vi "prueba5lector.vi"() -> ()   [LabVIEW 2012]
panel:
  out "Array":T1(array[cluster]) {"tanque3" scale=0.0..10.0; "tanque2" scale=0.0..10.0; "tanque1" scale=0.0..10.0}
  # "Elaborar un programa para adicionar este cluster a un archivo de texto.\nLuego debera hacer otro programa donde lea la informacion del archivo \nde texto y lo coloque en el cluster."
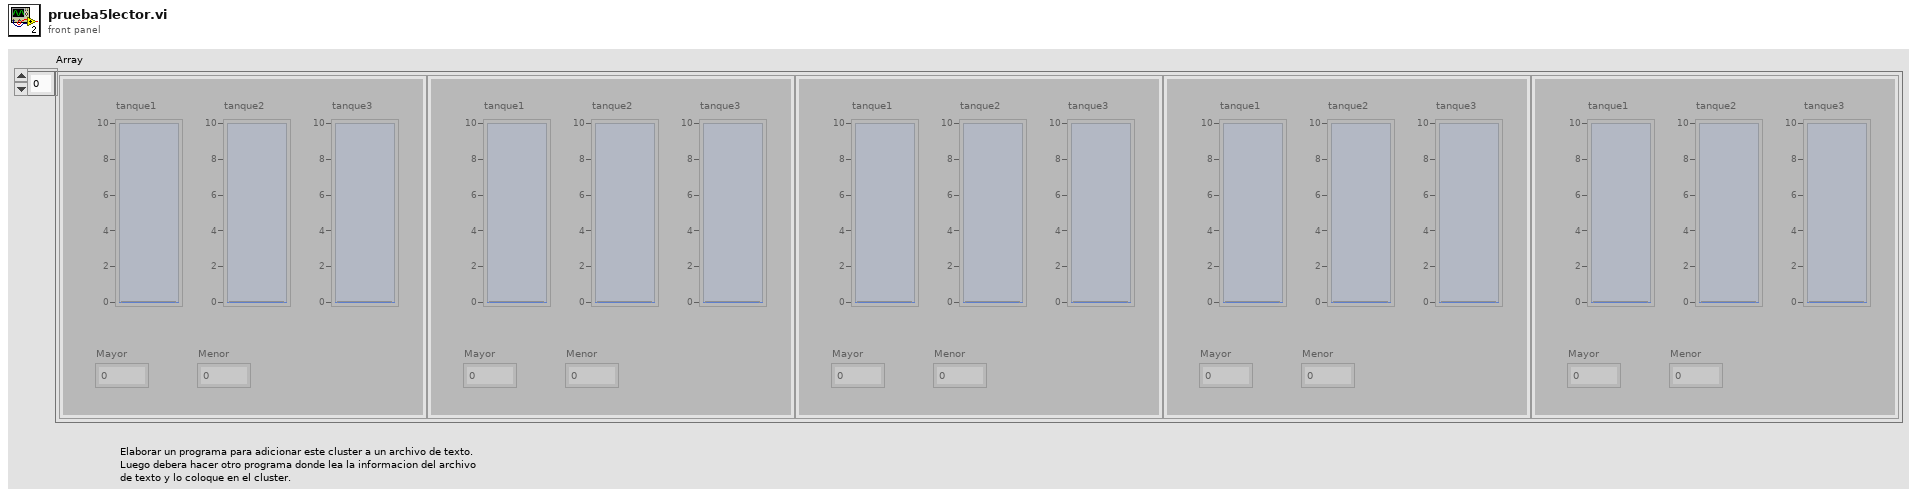
[diagram p1: front panel]
types:
  T1 = cluster{"tanque1":i32, "tanque2":i32, "tanque3":i32, "Mayor":dbl, "Menor":dbl}[]
  T2 = enum16{"open", "replace", "create", "open or create", "replace or create", "replace or create with confirmation"}
  T3 = cluster{"tanque1":i32, "tanque2":i32, "tanque3":i32, "Mayor":dbl, "Menor":dbl}
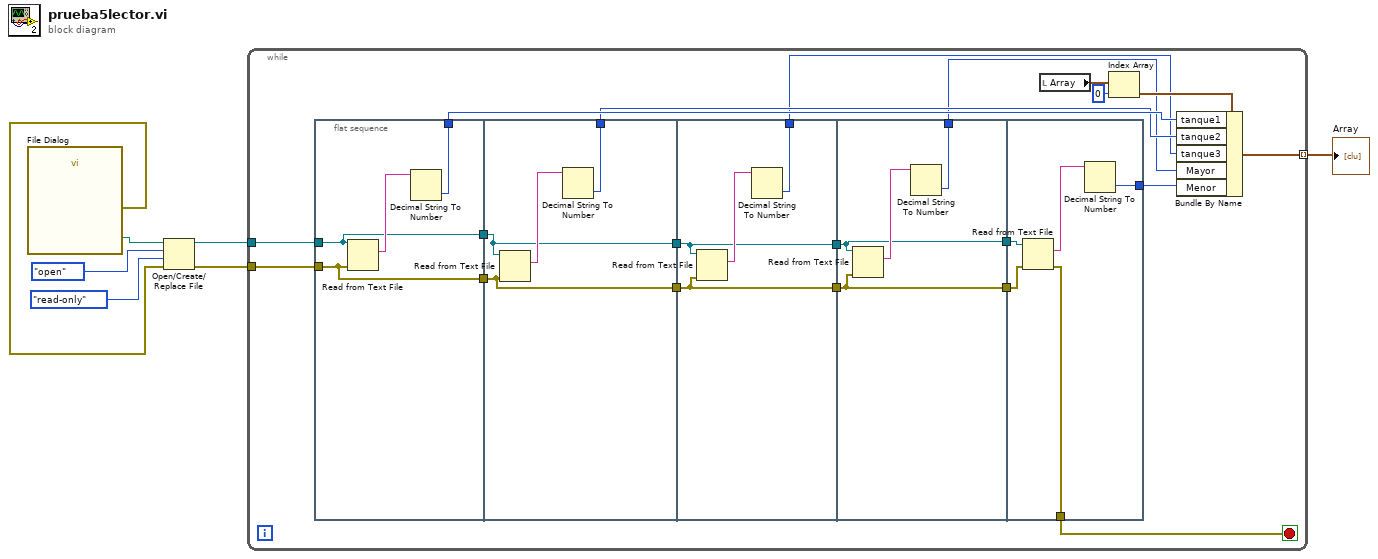
[diagram p0: block diagram]
diagram:
  n1 = call "File Dialog"() -> ("selected path"=w7:path, "error out"=w6:errorcluster)  [unwired: 12 in, 2 out]
  n2 = Open/Create/Replace File(file path (use dialog)=w7, error in=w6, operation (0:open)=T2."open", access (0:read/write)=enum16{"read/write", "read-only", "write-only"}."read-only") -> (refnum out=w3:refnum<file>, error out=w2:errorcluster)  [unwired: 2 in, 1 out]
  n3 = while {
    tunnel: w3 -> [w27]
    tunnel: w2 -> [w26]
    tunnel: [w8] -> w1 mode=indexing
    stop <- w17 stop-if-true
    n4 = flat-sequence {
      tunnel: w27 -> [w29]
      tunnel: w26 -> [w30]
      tunnel: [w30] -> w25
      tunnel: [w29] -> w24
      tunnel: [w28] -> w13
      tunnel: w25 -> [w34]
      tunnel: w24 -> [w33]
      tunnel: [w34] -> w23
      tunnel: [w33] -> w22
      tunnel: [w32] -> w12
      tunnel: w23 -> [w38]
      tunnel: w22 -> [w37]
      tunnel: [w38] -> w21
      tunnel: [w37] -> w20
      tunnel: [w36] -> w11
      tunnel: w21 -> [w42]
      tunnel: w20 -> [w41]
      tunnel: [w42] -> w19
      tunnel: [w41] -> w18
      tunnel: [w40] -> w10
      tunnel: w19 -> [w48]
      tunnel: w18 -> [w47]
      tunnel: [w45] -> w17
      tunnel: [w44] -> w9
      frame #0 {
        n5 = Read from Text File(file (use dialog)=w29, error in=w30) -> (text=w31:string)  [unwired: 2 in, 3 out]
        n6 = Decimal String To Number(string=w31) -> (number=w28:i32)  [unwired: 2 in, 1 out]
      }
      frame #1 {
        n7 = Read from Text File(file (use dialog)=w33, error in=w34) -> (text=w35:string)  [unwired: 2 in, 3 out]
        n8 = Decimal String To Number(string=w35) -> (number=w32:i32)  [unwired: 2 in, 1 out]
      }
      frame #2 {
        n9 = Read from Text File(file (use dialog)=w37, error in=w38) -> (text=w39:string)  [unwired: 2 in, 3 out]
        n10 = Decimal String To Number(string=w39) -> (number=w36:i32)  [unwired: 2 in, 1 out]
      }
      frame #3 {
        n11 = Read from Text File(file (use dialog)=w41, error in=w42) -> (text=w43:string)  [unwired: 2 in, 3 out]
        n12 = Decimal String To Number(string=w43) -> (number=w40:i32)  [unwired: 2 in, 1 out]
      }
      frame #4 {
        n13 = Read from Text File(file (use dialog)=w47, error in=w48) -> (text=w46:string, error out=w45:errorcluster)  [unwired: 2 in, 2 out]
        n14 = Decimal String To Number(string=w46) -> (number=w44:i32)  [unwired: 2 in, 1 out]
      }
    }
    n15 = local read "Array"() -> (w16:T1)
    n16 = Index Array(array=w16, index=0) -> (element=w14:T3)
    n17 = Bundle By Name(cluster=w14, "tanque1"=w13, "tanque2"=w12, "tanque3"=w11, "Mayor"=w10, "Menor"=w9) -> (w8:T3)
  }
  "Array" <- w1
